vi "type.property.set.vi"   [LabVIEW 2020]
uses:
  type.lvclass
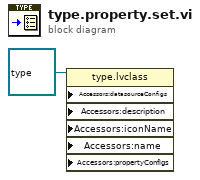
[diagram p0: block diagram]
diagram:
  n1 = property class="type.lvclass" props=["Accessors:datasourceConfigs", "Accessors:description", "Accessors:iconName", "Accessors:name", "Accessors:propertyConfigs"](reference=refnum<class "type.lvclass"> refnum ("type.lvclass")) -> ()  [unwired: 6 in, 2 out]
